vi "get folder total size.vi"(8 "error in (no error)":errorcluster, 10 "remote path":string, 11 "Refnum in":T1) -> (0 "error out":errorcluster, 2 "size":u64, 3 "Refnum out":T1)   [LabVIEW 2020]
uses:
  <vilib>/WebDAVClient/Advanced/SessionHandle.ctl
  <vilib>/WebDAVClient/NI_WebDAV.lvlib
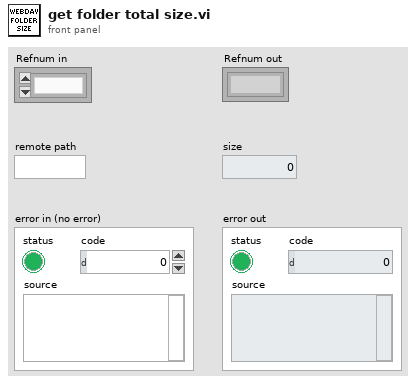
[diagram p1: front panel]
types:
  T1 = typedef "NI_WebDAV.lvlib/SessionHandle.ctl" = refnum<k1>
  T2 = typedef "NI_WebDAV.lvlib/FileInfo.ctl" = cluster{"type":string, "size":u64, "last modification":timestamp, "display name":string, "uri":string}
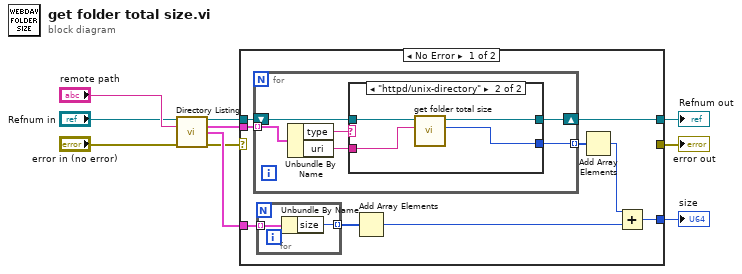
[diagram p0: block diagram]
diagram:
  n1 = call <vilib>:"Directory Listing.vi"("session handle"="Refnum in", "relative uri"="remote path", "error in (no error)"="error in (no error)") -> ("session handle out"=w4:T1, "directory list"=w3:T2[], "file list"=w8:T2[], "error out"=w7:errorcluster)  [unwired: 9 in]
  n2 = case shown="No Error" w7 {
    selector: w7 -> [_ w33]
    tunnel: w3 -> [w19 _]
    tunnel: w4 -> [w18 w34]
    tunnel: [w17 w34] -> w5
    tunnel: w8 -> [w15 _]
    tunnel: [_ w33] -> w9
    tunnel: [w13 _] -> w10
    frame No Error {
      n3 = for {
        tunnel: w19 -> [w27] mode=indexing
        shift-right: [w23] -> w17
        shift-left: w18 -> [w24]
        tunnel: [w22] -> w11 mode=indexing
        n4 = Unbundle By Name(w27) -> ("type"=w26:string, "uri"=w25:string)
        n5 = case shown="\"httpd/unix-directory\"" w26 {
          tunnel: w25 -> [_ w30]
          tunnel: w24 -> [w28 w32]
          tunnel: [w28 w31] -> w23
          tunnel: [_ w29] -> w22
          frame Default {
          }
          frame "httpd/unix-directory" {
            n6 = call "get folder total size.vi"("remote path"=w30, "Refnum in"=w32) -> ("size"=w29:u64, "Refnum out"=w31:T1)  [unwired: 7 in, 1 out]
          }
        }
      }
      n7 = for {
        tunnel: w15 -> [w21] mode=indexing
        tunnel: [w20] -> w16 mode=indexing
        n8 = Unbundle By Name(w21) -> ("size"=w20:u64)
      }
      n9 = Add Array Elements(numeric array=w16) -> (sum=w14:u64)
      n10 = Add Array Elements(numeric array=w11) -> (sum=w12:u64)
      n11 = Add(x=w12, y=w14) -> (x+y=w13:u64)
    }
    frame Error {
    }
  }
  "size" <- w10
  "error out" <- w9
  "Refnum out" <- w5
